vi "TRAJECTORY_EXECUTE_SWERVE.vi"(4 "Time Offset":dbl=-1.0 format="%16.4f", 6 "EnableClosedLoop":bool=TRUE, 8 "Init":bool, 9 "Reverse":bool, 10 "Follow Orientation":bool, 11 "Gyro Heading\nRAD":dbl) -> (0 "AtReference":bool, 1 "OutputTRAJ_STATE":T6={"TimeSeconds"=0.0, "Velocity"=0.0, "Acceleration"=0.0, "POSE"={"TRANSLATION"={"X"=0.0, "Y"=0.0}, "ROTATION"={"VALUE"=0.0, "COS"=1.0, "SIN"=0.0}}, "Curvature"=0.0} {"POSE"."ROTATION"."SIN" format="%13.4f"; "POSE"."ROTATION"."COS" format="%13.4f"; "POSE"."ROTATION"."VALUE" format="%13.4f"; "POSE"."TRANSLATION"."Y" format="%14.3f"; "POSE"."TRANSLATION"."X" format="%14.3f"}, 2 "Error and Corr":T4 {"Error Pose"."ROTATION"."SIN" format="%13.4f"; "Error Pose"."ROTATION"."COS" format="%13.4f"; "Error Pose"."ROTATION"."VALUE" format="%13.4f"; "Error Pose"."TRANSLATION"."Y" format="%14.3f"; "Error Pose"."TRANSLATION"."X" format="%14.3f"}, 3 "Chassis Velocity Target":T5 {"vOmega" format="%10.3f"; "vY" format="%10.3f"; "vX" format="%10.3f"}, 5 "Orientation Target":dbl)   [LabVIEW 2019]
uses:
  <vilib>/Rock Robotics/WPI/ThirdParty/JAS_Junk/TrajLib/Trajectory_Library.lvlib
  <vilib>/Rock Robotics/WPI/ThirdParty/JAS_Junk/TrajLib/TypeDef/TRANSLATION2D.ctl
  <vilib>/Rock Robotics/WPI/ThirdParty/JAS_Junk/TrajLib/TypeDef/ROTATION2D.ctl
  <vilib>/Rock Robotics/WPI/ThirdParty/JAS_Junk/TrajLib/TypeDef/POSE2D.ctl
  <vilib>/Rock Robotics/WPI/ThirdParty/JAS_Junk/TrajLib/TypeDef/TRAJ_STATE.ctl
  <vilib>/Rock Robotics/WPI/ThirdParty/JAS_Junk/TrajLib/TypeDef/CHASSIS_SPEEDS.ctl
panel:
  # "(FOR TESTING)"
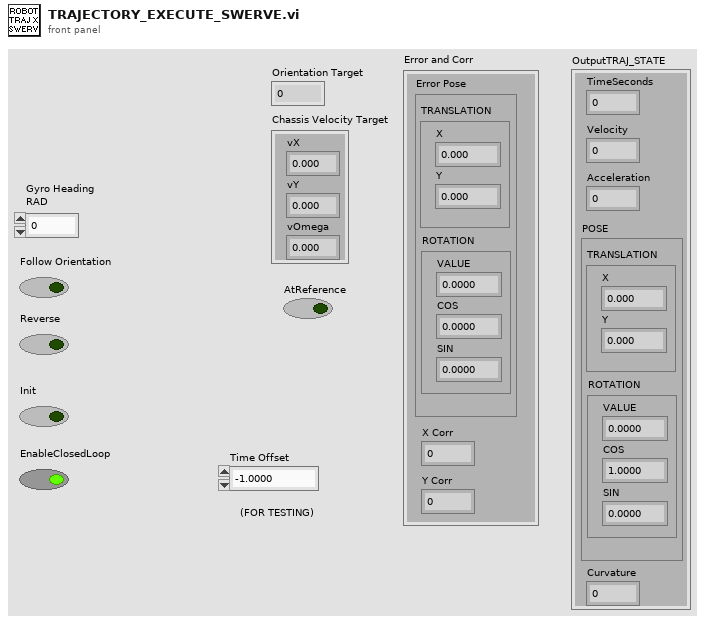
[diagram p1: front panel]
types:
  T1 = typedef "Trajectory_Library.lvlib/POSE2D.ctl" = cluster{"TRANSLATION":T2, "ROTATION":T3}
  T2 = typedef "Trajectory_Library.lvlib/TRANSLATION2D.ctl" = cluster{"X":dbl, "Y":dbl}
  T3 = typedef "Trajectory_Library.lvlib/ROTATION2D.ctl" = cluster{"VALUE":dbl, "COS":dbl, "SIN":dbl}
  T4 = cluster{"Error Pose":T1, "X Corr":dbl, "Y Corr":dbl}
  T5 = typedef "Trajectory_Library.lvlib/CHASSIS_SPEEDS.ctl" = cluster{"vX":dbl, "vY":dbl, "vOmega":dbl}
  T6 = typedef "Trajectory_Library.lvlib/TRAJ_STATE.ctl" = cluster{"TimeSeconds":dbl, "Velocity":dbl, "Acceleration":dbl, "POSE":T1, "Curvature":dbl}
  T7 = typedef "Trajectory_Library.lvlib/SWERVE_DRIVE_KINEMATICS.ctl" = cluster{"NumModules":i32, "InverseKinematics":T8, "ForwardKinematics":T8, "Modules":T2[], "PrevCoR":T2, "SavedModuleStates":T9[]}
  T8 = typedef "NI_Matrix.lvlib/RealMatrix.ctl" = dbl[][]
  T9 = typedef "Trajectory_Library.lvlib/SWERVE_DRIVE_MODULE_STATE.ctl" = cluster{"Speed":dbl, "Angle":T3}
  T10 = typedef "Trajectory_Library.lvlib/SWERVE_DRIVE_ODOMETRY.ctl" = cluster{"POSE":T1, "GyroOffset":T3, "PreviousAngle":T3, "PrevModulePositions":T11[], "NumModules":i32}
  T11 = typedef "Trajectory_Library.lvlib/SWERVE_DRIVE_MODULE_POSITION.ctl" = cluster{"Distance":dbl, "Angle":T3, "P":bool}
  T12 = typedef "Trajectory_Library.lvlib/TRAJECTORY.ctl" = cluster{"TotalTImeSecs":dbl, "States":T6[]}
  T13 = typedef "Trajectory_Library.lvlib/PID_TUNING.ctl" = cluster{"Kp":dbl, "Ki":dbl, "Kd":dbl, "MaximumIntegral":dbl, "MinimumIntegral":dbl}
  T14 = typedef "Trajectory_Library.lvlib/PROFILED_PID_CONTROLLER.ctl" = cluster{"Controller":T15, "Goal":T16, "Setpoint":T16, "Constraint":T17}
  T15 = typedef "Trajectory_Library.lvlib/PID_CONTROLLER.ctl" = cluster{"Kp":dbl, "Ki":dbl, "Kd":dbl, "Period":dbl, "Max_Integral":dbl, "Min_Integral":dbl, "Max_Input":dbl, "Min_Input":dbl, "Continuous":bool, "PositionError":dbl, "VelocityError":dbl, "PrevError":dbl, "TotalError":dbl, "PositionTolerance":dbl, "VelocityTolerance":dbl, "SetPoint":dbl, "Kf":dbl, "Prev_Deriv":dbl, "Prev_Deriv 2":dbl, "DerivativeFilter":bool, "Min_Output":dbl, "Max_Output":dbl, "Prev_F_P":dbl, "Prev_F_P_2":dbl, "AntiWindupActive":bool, "Measurement":dbl}
  T16 = typedef "Trajectory_Library.lvlib/TRAPEZOID_PROFILE_STATE.ctl" = cluster{"Position":dbl, "Velocity":dbl}
  T17 = typedef "Trajectory_Library.lvlib/TRAPEZOID_PROFILE_CONSTRAINT.ctl" = cluster{"MaxVelocity":dbl, "MaxAcceleration":dbl}
  T18 = typedef "Trajectory_Library.lvlib/HOLONOMIC_DRV_CTRL.ctl" = cluster{"poseTolerance":T1, "poseError":T1, "Enabled":bool, "PID_xCtrl":T15, "PID_yCtrl":T15, "PROF_PID_thetaCtrl":T14, "RotationError":T3, "FirstRun":bool}
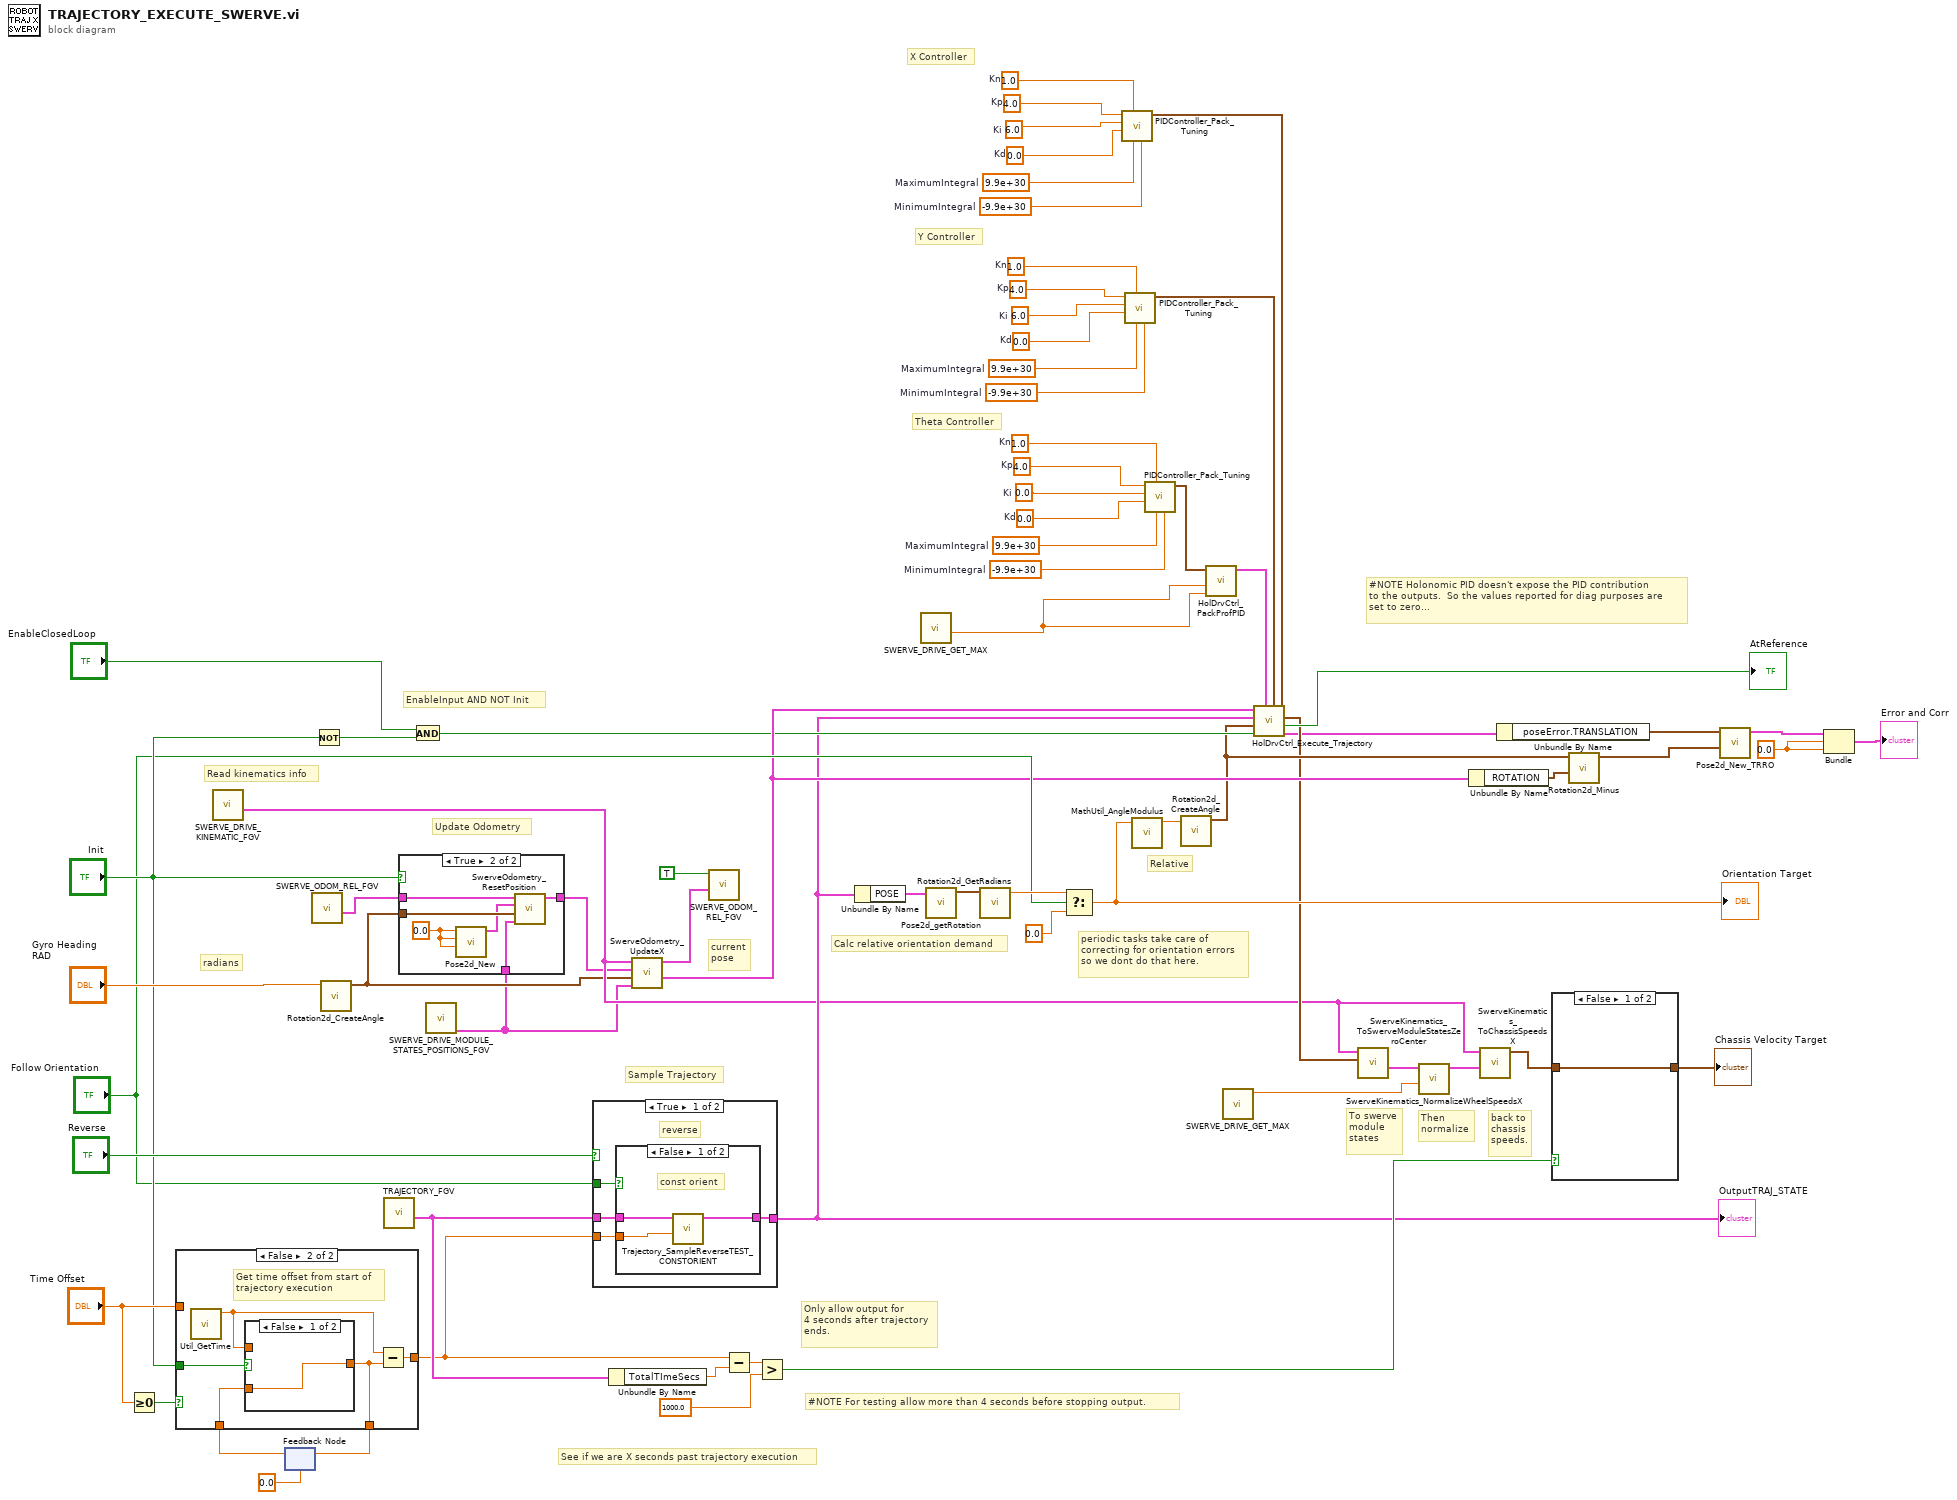
[diagram p0: block diagram]
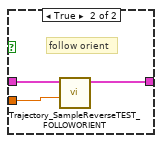
[diagram p4: hidden frame]
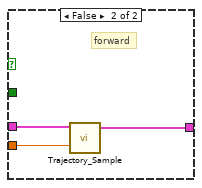
[diagram p5: hidden frame]
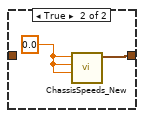
[diagram p7: hidden frame]
diagram:
  w20 = 1.0  # Kn
  w23 = 4.0  # Kp
  w32 = 0.0  # Ki
  w33 = 0.0  # Kd
  w34 = 9.9e+30  # MaximumIntegral
  w35 = -9.9e+30  # MinimumIntegral
  w18 = 1.0  # Kn
  w21 = 4.0  # Kp
  w24 = 6.0  # Ki
  w25 = 0.0  # Kd
  w26 = 9.9e+30  # MaximumIntegral
  w27 = -9.9e+30  # MinimumIntegral
  w19 = 1.0  # Kn
  w22 = 4.0  # Kp
  w28 = 6.0  # Ki
  w29 = 0.0  # Kd
  w30 = 9.9e+30  # MaximumIntegral
  w31 = -9.9e+30  # MinimumIntegral
  w47 = 0.0
  # "#NOTE For testing allow more than 4 seconds before stopping output."
  # "EnableInput AND NOT Init"
  # "Theta Controller"
  # "Y Controller"
  # "X Controller"
  # "Relative"
  # "#NOTE Holonomic PID doesn't expose the PID contribution \nto the outputs.  So the values reported for diag purposes are\nset to zero..."
  # "current\npose"
  # "back to\nchassis\nspeeds."
  # "Then\nnormalize"
  # "To swerve\nmodule\nstates"
  # "Calc relative orientation demand"
  # "Read kinematics info"
  # "Sample Trajectory"
  # "See if we are X seconds past trajectory execution"
  # "Update Odometry"
  # "radians"
  # "periodic tasks take care of\ncorrecting for orientation errors\nso we dont do that here."
  # "Only allow output for\n4 seconds after trajectory\nends."
  n1 = Greater Or Equal To 0?(x="Time Offset") -> (x >= 0?=w51:bool)
  n2 = call "SWERVE_DRIVE_KINEMATIC_FGV.vi"() -> ("out SWERVE_DRIVE_KINEMATICS"=w5:T7)  [unwired: 11 in]
  n3 = feedback #1(0.0 ("TIME")) -> (w53:dbl)
  n4 = case shown="False" w51 {
    tunnel: [w72 w78] -> w69
    tunnel: "Init" -> [_ w76]
    tunnel: w53 -> [w73 w75]
    tunnel: [w73 w74] -> w52
    tunnel: "Time Offset" -> [w72 _]
    frame True {
      # "For testing allow\nuser entered time offset!!"
    }
    frame False {
      # "Get time offset from start of\ntrajectory execution"
      n5 = call <vilib>:"Util_GetTime.vi"() -> ("FPGA_Time_Seconds"=w77:dbl)  [unwired: 10 in, 1 out]
      n6 = case shown="False" w76 {
        tunnel: [w79 w80] -> w74
        tunnel: w75 -> [w79 _]
        tunnel: w77 -> [_ w80]
        frame False {
        }
        frame True {
        }
      }
      n7 = Subtract(x=w77, y=w74) -> (x-y=w78:dbl)
    }
  }
  n8 = feedback-in #1(w52) -> ()
  n9 = call "SWERVE_ODOM_REL_FGV.vi"() -> ("out SWERVE_DRIVE_ODOMETRY"=w64:T10)  [unwired: 11 in]
  n10 = Not(x="Init") -> (.not. x?=w48:bool)
  n11 = call <vilib>:"Rotation2d_CreateAngle.vi"("Angle"="Gyro Heading\nRAD") -> ("ROTATION"=w3:T3)  [unwired: 10 in]
  n12 = call "TRAJECTORY_FGV.vi"() -> ("outTRAJECTORY"=w71:T12)  [unwired: 11 in]
  n13 = And(x="EnableClosedLoop", y=w48) -> (x .and. y?=w11:bool)
  n14 = call "SWERVE_DRIVE_MODULE_STATES_POSITIONS_FGV.vi"() -> ("out Current Module Positions"=w2:T11[])  [unwired: 10 in, 1 out]
  n15 = case shown="True" "Init" {
    tunnel: w64 -> [w81 w87]
    tunnel: [w81 w86] -> w4
    tunnel: w3 -> [_ w85]
    tunnel: w2 -> [_ w82]
    frame False {
    }
    frame True {
      w84 = 0.0 ("X")
      n16 = call <vilib>:"Pose2d_New.vi"("Heading"=w84, "Y"=w84, "X"=w84) -> ("out POSe"=w83:T1)  [unwired: 8 in]
      n17 = call <vilib>:"SwerveOdometry_ResetPosition.vi"("Module Positions"=w82, "gyroAngle"=w85, "Pose"=w83, "in SWERVE_DRIVE_ODOMETRY"=w87) -> ("out SWERVE_DRIVE_ODOMETRY"=w86:T10)  [unwired: 6 in, 1 out]
    }
  }
  n18 = case shown="True" "Reverse" {
    tunnel: w71 -> [w91 w100]
    tunnel: w69 -> [w89 w99]
    tunnel: [w90 w98] -> w10
    tunnel: "Follow Orientation" -> [w88 _]
    frame True {
      # "reverse"
      n19 = case shown="False" w88 {
        tunnel: w91 -> [w94 w97]
        tunnel: [w92 w96] -> w90
        tunnel: w89 -> [w93 w95]
        frame False {
          # "const orient"
          n20 = call "Trajectory_SampleReverseTEST_CONSTORIENT.vi"("Time"=w93, "InputTRAJECTORY"=w94) -> ("OutputTRAJ_STATE"=w92:T6)  [unwired: 9 in]
        }
        frame True {
          # "follow orient"
          n21 = call "Trajectory_SampleReverseTEST_FOLLOWORIENT.vi"("Time"=w95, "InputTRAJECTORY"=w97) -> ("OutputTRAJ_STATE"=w96:T6)  [unwired: 9 in]
        }
      }
    }
    frame False {
      # "forward"
      n22 = call <vilib>:"Trajectory_Sample.vi"("Time"=w99, "InputTRAJECTORY"=w100) -> ("OutputTRAJ_STATE"=w98:T6)  [unwired: 9 in]
    }
  }
  "OutputTRAJ_STATE" <- w10
  n23 = Unbundle By Name(w71) -> ("TotalTImeSecs"=w70:dbl)
  n24 = call <vilib>:"SwerveOdometry_UpdateX.vi"("module Positions"=w2, "gyroAngle"=w3, "in SWERVE_DRIVE_ODOMETRY"=w4, "SWERVE_DRIVE_KINEMATICS"=w5) -> ("robot POSE"=w12:T1, "out SWERVE_DRIVE_ODOMETRY"=w58:T10)  [unwired: 5 in, 1 out]
  n25 = call "SWERVE_ODOM_REL_FGV.vi"("in SWERVE_DRIVE_ODOMETRY"=w58, "WRITE"=TRUE) -> ()  [unwired: 9 in, 1 out]
  n26 = Subtract(x=w69, y=w70) -> (x-y=w68:dbl)
  n27 = Greater?(x=w68, y=1000.0) -> (0:w66:bool)
  n28 = Unbundle By Name(w10) -> ("POSE"=w55:T1)
  n29 = call "SWERVE_DRIVE_GET_MAX.vi"() -> ("Max Rotational Vel (Rad/Sec)"=w13:dbl)  [unwired: 10 in, 1 out]
  n30 = call <vilib>:"Pose2d_getRotation.vi"("in POSE"=w55) -> ("out ROTATION"=w60:T3)  [unwired: 10 in]
  n31 = call <vilib>:"Rotation2d_GetRadians.vi"("in ROTATION"=w60) -> ("AngleRadians"=w39:dbl)  [unwired: 10 in]
  n32 = Select(t=w39, s="Follow Orientation", f=0.0) -> (s? t:f=w36:dbl)
  "Orientation Target" <- w36
  n33 = call <vilib>:"PIDController_Pack_Tuning.vi"("MinimumIntegral"=w27, "MaximumIntegral"=w26, "Kn"=w18, "Kd"=w25, "Ki"=w24, "Kp"=w21) -> ("PID Tuning"=w14:T13)  [unwired: 5 in]
  n34 = call <vilib>:"PIDController_Pack_Tuning.vi"("MinimumIntegral"=w31, "MaximumIntegral"=w30, "Kn"=w19, "Kd"=w29, "Ki"=w28, "Kp"=w22) -> ("PID Tuning"=w15:T13)  [unwired: 5 in]
  n35 = call <vilib>:"MathUtil_AngleModulus.vi"("InputAngle"=w36) -> ("ModulsAngle"=w45:dbl)  [unwired: 10 in]
  n36 = call <vilib>:"PIDController_Pack_Tuning.vi"("MinimumIntegral"=w35, "MaximumIntegral"=w34, "Kn"=w20, "Kd"=w33, "Ki"=w32, "Kp"=w23) -> ("PID Tuning"=w17:T13)  [unwired: 5 in]
  n37 = call <vilib>:"Rotation2d_CreateAngle.vi"("Angle"=w45) -> ("ROTATION"=w9:T3)  [unwired: 10 in]
  n38 = call <vilib>:"HolDrvCtrl_PackProfPID.vi"("Max Accel"=w13, "Max Speed"=w13, "Theta PID Tuning"=w17) -> ("Theta PID CONTROLLER"=w16:T14)  [unwired: 8 in]
  n39 = call "SWERVE_DRIVE_GET_MAX.vi"() -> ("Max Wheel Vel (Meter/Sec)"=w56:dbl)  [unwired: 10 in, 1 out]
  n40 = call <vilib>:"HolDrvCtrl_Execute_Trajectory.vi"("X PID Tuning"=w14, "Y PID Tuning"=w15, "thetaProfiledPID_CTRL"=w16, "Enable"=w11, "angleRef"=w9, "desiredTrajState"=w10, "currentPose"=w12) -> ("outHOLONOMIC_DRV_CTRL"=w6:T18, "AtReference"=→"AtReference":bool, "calcChassisSpeed"=w7:T5)  [unwired: 2 in]
  n41 = call <vilib>:"SwerveKinematics_ToSwerveModuleStatesZeroCenter.vi"("ChassisSpeeds"=w7, "in SWERVE_DRIVE_KINEMATICS"=w5) -> ("ModuleStates"=w62:T9[])  [unwired: 8 in, 1 out]
  n42 = call <vilib>:"SwerveKinematics_NormalizeWheelSpeedsX.vi"("AttainableMaxSpeed"=w56, "in WheelStates"=w62) -> ("out WheelStates"=w61:T9[])  [unwired: 9 in]
  n43 = Unbundle By Name(w12) -> ("ROTATION"=w40:T3)
  n44 = call <vilib>:"SwerveKinematics_ToChassisSpeedsX.vi"("WheelStates"=w61, "in SWERVE_DRIVE_KINEMATICS"=w5) -> ("Chassis Speed"=w1:T5)  [unwired: 9 in]
  n45 = Unbundle By Name(w6) -> ("poseError.TRANSLATION"=w44:T2)
  n46 = case shown="False" w66 {
    tunnel: w1 -> [w101 _]
    tunnel: [w101 w102] -> w57
    frame False {
    }
    frame True {
      w103 = 0.0 ("vX")
      n47 = call <vilib>:"ChassisSpeeds_New.vi"("vAngular"=w103, "vY"=w103, "vX"=w103) -> ("CHASSIS"=w102:T5)  [unwired: 8 in]
    }
  }
  "Chassis Velocity Target" <- w57
  n48 = call <vilib>:"Rotation2d_Minus.vi"("other ROTATION"=w40, "in ROTATION"=w9) -> ("out ROTATION"=w43:T3)  [unwired: 9 in]
  n49 = call <vilib>:"Pose2d_New_TRRO.vi"("ROTATION"=w43, "TRANSLATION"=w44) -> ("outPOSE"=w42:T1)  [unwired: 9 in]
  n50 = Bundle("outPOSE"=w42, w47, w47) -> (→"Error and Corr":cluster{"outPOSE":T1, dbl, dbl})  [unwired: 1 in]
